vi "QtoMdotConvertor.vi"() -> ()   [LabVIEW 2016]
uses:
  Anemometry Sub Vis/Controls/GasCombo.ctl
panel:
  in  "Tab Control":enum32{"QtoMdot", "Cal To ADAM"}(tab)
  in  "Cal Gas":T1
  in  "Voume flowrate":dbl format="%#_g l/min"
  out "Mass flowrate":dbl format="%#_g g/min"
  in  "CalibrationA":dbl
  in  "CalibrationB":dbl
  in  "SpanX (C)":dbl
  in  "ZeroX (A)":dbl
  out "SpanY (D)":dbl
  out "ZeroY (B)":dbl
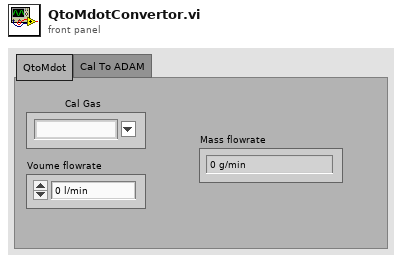
[diagram p1: front panel]
types:
  T1 = typedef "GasCombo.ctl" = string
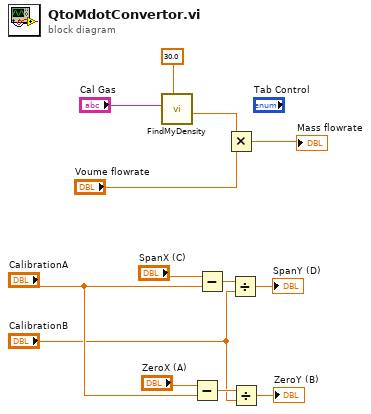
[diagram p0: block diagram]
diagram:
  n1 = call "FindMyDensity.vi"("History (s)"=30.0, "Cal Gas"="Cal Gas") -> ("Density"=w11:dbl)  [unwired: 9 in]
  n2 = Subtract(x="ZeroX (A)", y="CalibrationA") -> (x-y=w3:dbl)
  n3 = Subtract(x="SpanX (C)", y="CalibrationA") -> (x-y=w7:dbl)
  n4 = Multiply(x=w11, y="Voume flowrate") -> (x*y=→"Mass flowrate":dbl)
  n5 = Divide(x=w7, y="CalibrationB") -> (x/y=→"SpanY (D)":dbl)
  n6 = Divide(x=w3, y="CalibrationB") -> (x/y=→"ZeroY (B)":dbl)
